vi "Delimited String to Key-Value Array.vi"(8 "error in (no error)":errorcluster, 10 "Delimited String":string) -> (0 "error out":errorcluster, 2 "Key/Value Pairs":cluster{"Key":string, "Value":string}[](array[cluster]))   [LabVIEW 2025, in "Interface Functions.lvlib"]
uses:
  <vilib>/Utility/error.llb/Trim Whitespace One-Sided.vi
  <vilib>/Utility/error.llb/Error Cluster From Error Code.vi
  <vilib>/ErrorRing/Error Ring.xnode
  Interface Functions/Interface Functions.lvlib
panel:
  # "key1=value1,key2=value2,key3=value3"
  # "Comma-separated key/value pairs separated by equals sign.\n\nKeys and values are converted to uppercase for better comparison."
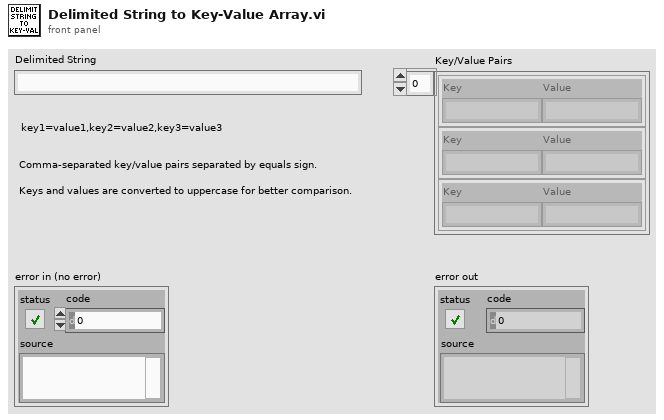
[diagram p1: front panel]
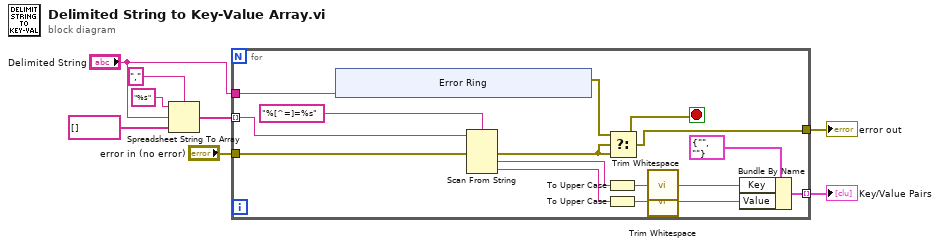
[diagram p0: block diagram]
diagram:
  n1 = Spreadsheet String To Array(delimiter (Tab)=",", format string="%s", spreadsheet string="Delimited String", array type (2D Dbl)=string[] []) -> (array=w5:string[])
  n2 = for {
    tunnel: w5 -> [w14] mode=indexing
    tunnel: [w21] -> w4 mode=indexing
    tunnel: "error in (no error)" -> [w18]
    tunnel: [w16] -> w3
    tunnel: "Delimited String" -> [w13]
    stop <- w16 stop-if-true
    n3 = xnode "Error Ring"("parameter 0"=w13) -> ("error out"=w15:errorcluster)
    n4 = Scan From String(format string="%[^=]=%s", input string=w14, error in=w18) -> (error out=w17:errorcluster, output 1=w19:string, output 2=w20:string)  [unwired: 3 in, 2 out]
    n5 = To Upper Case(1:w19) -> (0:w12:string)
    n6 = To Upper Case(1:w20) -> (0:w11:string)
    n7 = Select(t=w15, s=w17, f=w17) -> (s? t:f=w16:errorcluster)
    n8 = call <vilib>:"Trim Whitespace.vi"("string"=w12) -> ("trimmed string"=w9:string)  [unwired: 1 in]
    n9 = call <vilib>:"Trim Whitespace.vi"("string"=w11) -> ("trimmed string"=w10:string)  [unwired: 1 in]
    n10 = Bundle By Name(cluster=cluster{"Key":string, "Value":string} {"Key"="", "Value"=""} ("Cluster"), "Key"=w9, "Value"=w10) -> (w21:cluster{"Key":string, "Value":string})
  }
  "Key/Value Pairs" <- w4
  "error out" <- w3
